vi "2ND_STAGE.vi"() -> (0 "Stage 2 Temperature":dbl(graph), 1 "Coolant Temperature":dbl, 2 "Pressure Transmitter":dbl, 3 "Stage 2 Coolant Temperature":dbl(graph), 4 "Stage 2 Pressure":dbl(graph), 5 "Temperature Transmitter":dbl)   [LabVIEW 2014]
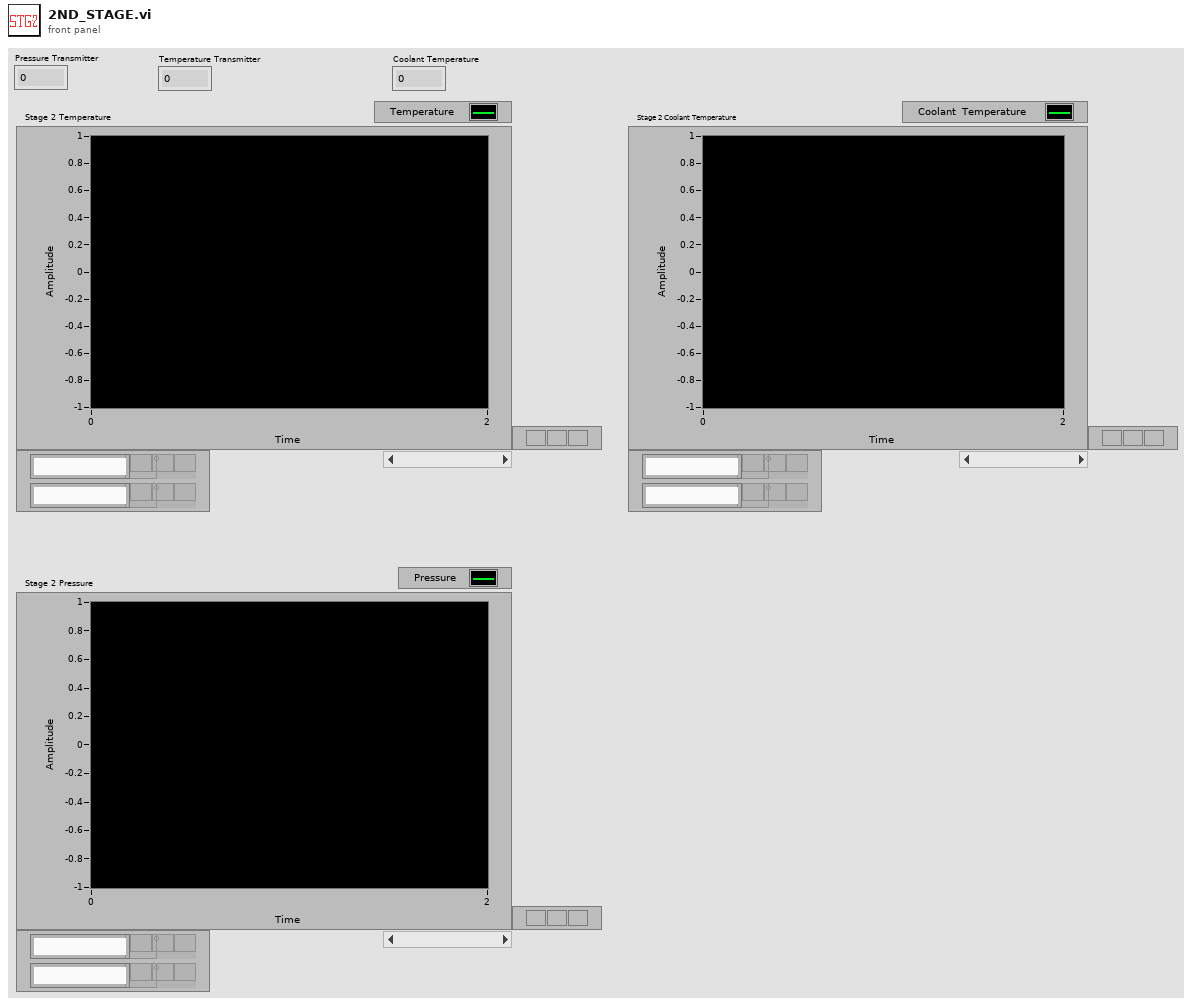
[diagram p1: front panel]
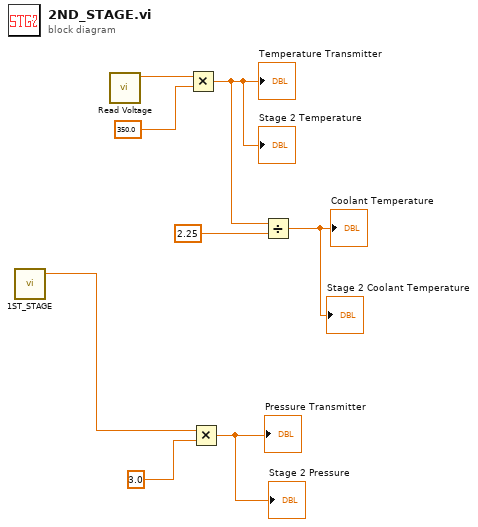
[diagram p0: block diagram]
diagram:
  n1 = call "1ST_STAGE.vi"() -> ("Pressure Transmitter"=w1:dbl)  [unwired: 5 out]
  n2 = call "Read Voltage.vi"() -> ("voltage"=w8:dbl)  [unwired: 6 in, 1 out]
  n3 = Multiply(x=w8, y=350.0) -> (x*y=w6:dbl)
  "Temperature Transmitter" <- w6
  "Stage 2 Temperature" <- w6
  n4 = Multiply(x=w1, y=3.0) -> (x*y=→"Pressure Transmitter" →"Stage 2 Pressure":dbl)
  n5 = Divide(x=w6, y=2.25) -> (x/y=→"Coolant Temperature" →"Stage 2 Coolant Temperature":dbl)
